vi "[PC]MainGUI_User.vi"() -> ()   [LabVIEW 2018]
uses:
  TypeDef/ControllerState.ctl
panel:
  in  "volume":dbl=70.0 format="%#_g ml"
  in  "Emg Stop":bool caption="STOP"
  out "Druck":dbl(slide) scale=0.0..30.0
  out "Temperatur":dbl(slide) scale=0.0..100.0
  in  "stop":bool
  in  "temp":dbl=70.0 format="%#_g °C"
  in  "Kaffee anfordern":bool
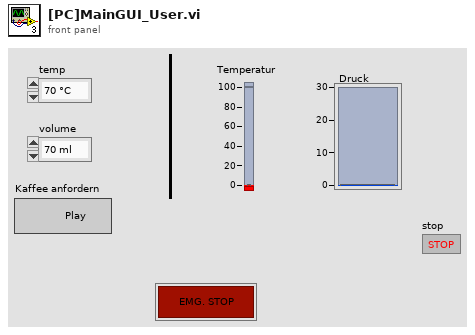
[diagram p1: front panel]
types:
  T1 = typedef "ControllerState.ctl" = enum16{"Idle", "Vorheizen", "Brühen", "Emergency-Stop"}
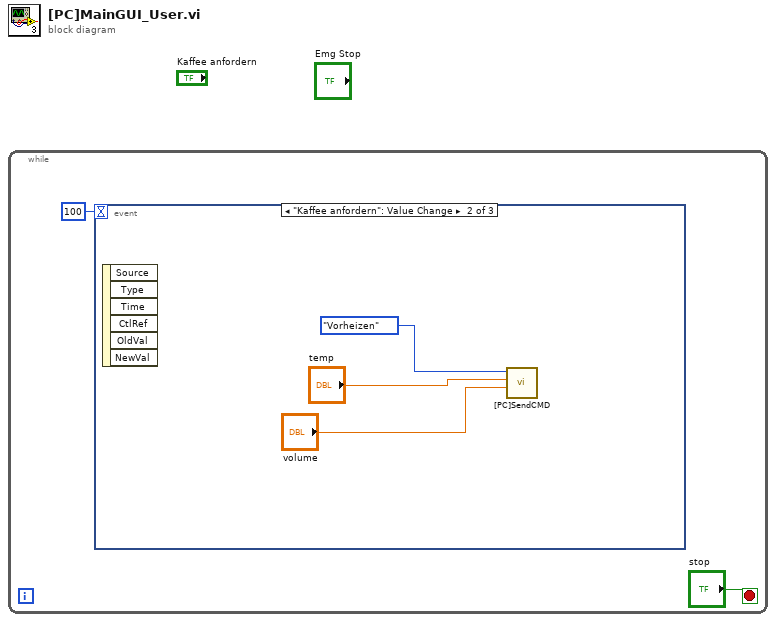
[diagram p0: block diagram]
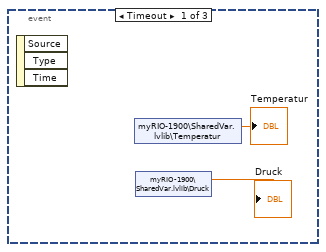
[diagram p2: hidden frame]
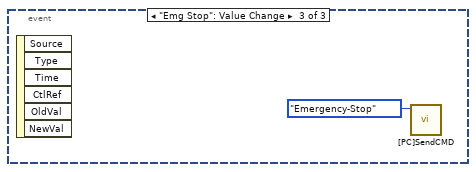
[diagram p3: hidden frame]
diagram:
  n1 = while {
    stop <- "stop" stop-if-true
    n2 = event shown="[1] \"Kaffee anfordern\": Value Change" {
      selector: _ -> [_ _ _]
      dyn-events: _ -> [_ _ _]
      timeout: 100 -> [_ _ _]
      event Timeout {
        n3 = event-data() -> ()  [unwired: 1 in, 3 out]
        n4 = shared-variable "myRIO-1900\\SharedVar.lvlib\\Temperatur"() -> (→"Temperatur":dbl)  [unwired: 1 in, 1 out]
        n5 = shared-variable "myRIO-1900\\SharedVar.lvlib\\Druck"() -> (→"Druck":dbl)  [unwired: 1 in, 1 out]
      }
      event "Kaffee anfordern": Value Change {
        n6 = event-data() -> ()  [unwired: 1 in, 6 out]
        n7 = call "[PC]SendCMD.vi"("volume"="volume", "temp"="temp", "State Rqst"=ControllerState."Vorheizen") -> ()  [unwired: 9 in]
      }
      event "Emg Stop": Value Change {
        n8 = event-data() -> ()  [unwired: 1 in, 6 out]
        n9 = call "[PC]SendCMD.vi"("State Rqst"=ControllerState."Emergency-Stop") -> ()  [unwired: 11 in]
      }
    }
  }
